vi "Throttle Multiplier.vi"(10 "Slider":dbl(slide) scale=0.0..1.0, 11 "Input":dbl) -> (3 "Output":dbl)   [LabVIEW 2016]
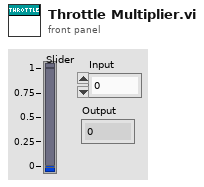
[diagram p1: front panel]
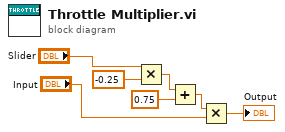
[diagram p0: block diagram]
diagram:
  n1 = Multiply(x="Slider", y=-0.25) -> (x*y=w7:dbl)
  n2 = Add(x=w7, y=0.75) -> (x+y=w1:dbl)
  n3 = Multiply(x=w1, y="Input") -> (x*y=→"Output":dbl)
